vi "Write and Read Multiple Registers.vi"(4 "read count":u16, 6 "read starting address":u16, 8 "error in":errorcluster, 9 "write values":u16[](array[numeric]), 10 "write starting address":u16, 11 "device data model in":refnum<class "Standard Data Model.lvclass">) -> (0 "error out":errorcluster, 1 "read values":u16[](array[numeric]), 3 "device data model out":refnum<class "Standard Data Model.lvclass">)   [LabVIEW 2021, in "Standard Data Model.lvclass"]
doc: "Writes and reads the values of multiple register values in series. The <b>write values</b> are inserted starting at <b>write starting address</b> and the returned <b>read values</b> consists of <b>read count</b> holding registers starting at <b>read starting address</b>."
uses:
  Standard Data Model.lvclass
  Standard Data Model.lvclass/Standard Data Model.ctl
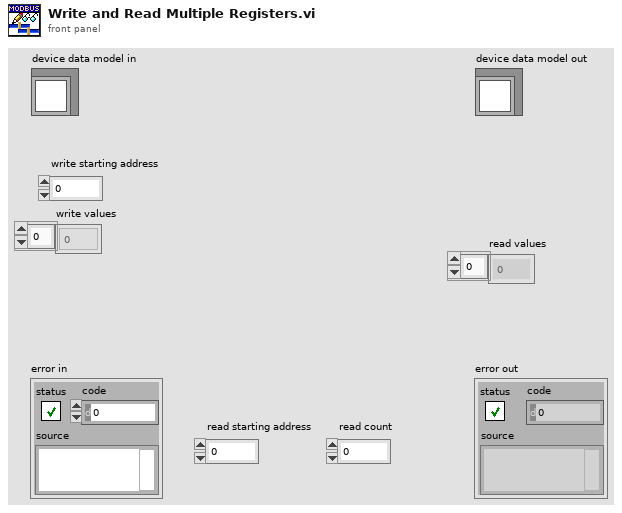
[diagram p1: front panel]
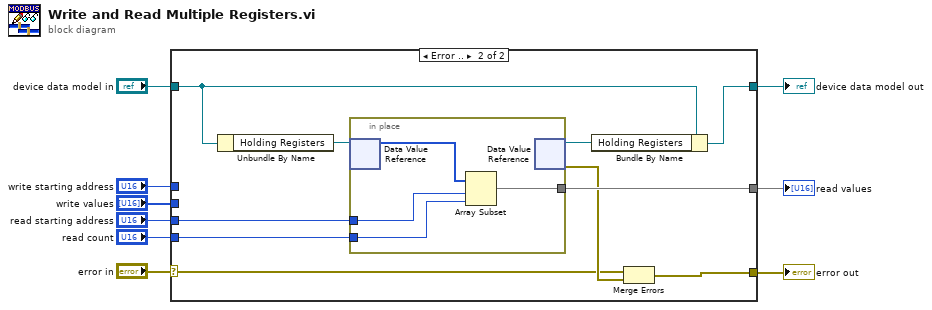
[diagram p0: block diagram]
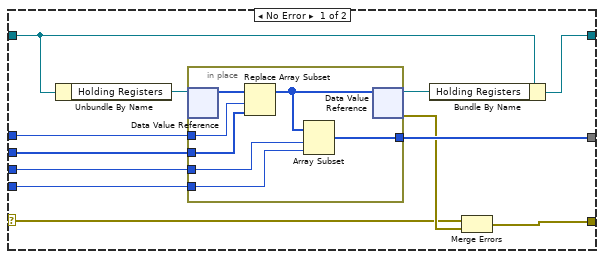
[diagram p2: hidden frame]
diagram:
  n1 = case shown="Error .." "error in" {
    selector: "error in" -> [w10 w29]
    tunnel: "device data model in" -> [w21 w38]
    tunnel: [w20 w37] -> w8
    tunnel: "write values" -> [w18 _]
    tunnel: "write starting address" -> [w17 _]
    tunnel: [w16 w35] -> w5
    tunnel: "read count" -> [w15 w34]
    tunnel: "read starting address" -> [w14 w33]
    tunnel: [w13 w32] -> w2
    frame No Error {
      n2 = Unbundle By Name(w21) -> ("Holding Registers"=w19:refnum<data-value>)
      n3 = in-place {
        in-place-border: w18 -> [w28]
        in-place-border: w17 -> [w27]
        in-place-border: [w24] -> w16
        in-place-border: w15 -> [w23]
        in-place-border: w14 -> [w22]
        n4 = in-place-dvr #1(w19) -> (w26:u16[])  [unwired: 1 out]
        n5 = Replace Array Subset(array=w26, new element=w28, index=w27) -> (w25:u16[])
        n6 = Array Subset(array=w25, index=w22, length=w23) -> (w24:u16[])
        n7 = in-place-dvr #1(w25) -> (w12:refnum<data-value>, w11:errorcluster)
      }
      n8 = Bundle By Name(cluster=w21, "Holding Registers"=w12) -> (w13:refnum<class "Standard Data Model.lvclass">)
      n9 = Merge Errors(w10, w11) -> (w20:errorcluster)
    }
    frame Error {
      n10 = Unbundle By Name(w38) -> ("Holding Registers"=w36:refnum<data-value>)
      n11 = in-place {
        in-place-border: [w42] -> w35
        in-place-border: w34 -> [w41]
        in-place-border: w33 -> [w40]
        n12 = in-place-dvr #2(w36) -> (w39:u16[])  [unwired: 1 out]
        n13 = Array Subset(array=w39, index=w40, length=w41) -> (w42:u16[])
        n14 = in-place-dvr #2() -> (w31:refnum<data-value>, w30:errorcluster)  [unwired: 1 in]
      }
      n15 = Bundle By Name(cluster=w38, "Holding Registers"=w31) -> (w32:refnum<class "Standard Data Model.lvclass">)
      n16 = Merge Errors(w29, w30) -> (w37:errorcluster)
    }
  }
  "error out" <- w8
  "device data model out" <- w2
  "read values" <- w5
